vi "HostSubViTest.vi"() -> ()   [LabVIEW 2014]
uses:
  <vilib>/rvi/interface/nirviOpenFPGA/nirviOpenFPGA.xnode
  <vilib>/rvi/interface/nirviReadWriteControl/nirviReadWriteControl.xnode
  <vilib>/rvi/interface/nirviCloseFPGA/nirviCloseFPGA.xnode
  FPGA Bitfiles/TiTaProj_DAF_SubViTestTopLeve_vbBMOXiu67U.lvbitx
  SubViTestTopLevel.vi
  <vilib>/FPGAPlugInAG/PXI-7852R/niLvFpga_Open_PXI-7852R.vi
  <vilib>/rvi/interface/common/dynamic/niFpgaDynamicAddResources.vi
  NiFpgaLv.dll
  <vilib>/Utility/error.llb/Error Cluster From Error Code.vi
  <vilib>/rvi/interface/Simulation/niFpgaSimulationCallBeginRW.vi
  <vilib>/rvi/errors/niLvFpgaAdjustHostInterfaceError.vi
  <vilib>/FPGAPlugInAG/Dynamic/niLvFpga_Close_Dynamic.vi
panel:
  in  "stop 2":bool
  in  "stop":bool
  out "0notPressed1Pressed":i16
  out "insideloop":i32
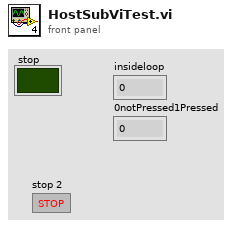
[diagram p1: front panel]
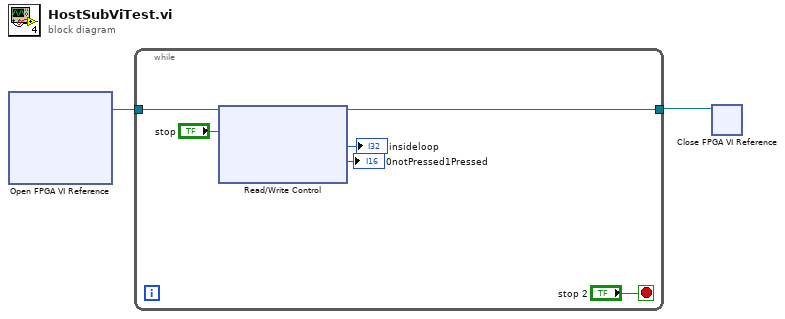
[diagram p0: block diagram]
diagram:
  n1 = xnode "Open FPGA VI Reference"() -> ("FPGA VI Reference Out"=w2:refnum<k20>)  [unwired: 2 in, 1 out]
  n2 = while {
    tunnel: w2 -> [w8]
    tunnel: [w3] -> w1
    stop <- "stop 2" stop-if-true
    n3 = xnode "Read/Write Control"("FPGA VI Reference In"=w8, "stop"="stop") -> ("FPGA VI Reference Out"=w3:refnum<k20>, "insideloop"=→"insideloop":i32, "0notPressed1Pressed"=→"0notPressed1Pressed":i16)  [unwired: 2 in, 1 out]
  }
  n4 = xnode "Close FPGA VI Reference"("FPGA VI Reference In"=w1) -> ()  [unwired: 1 in, 1 out]
